vi "LoadObjects_LookupTable.vi"(6 "UIMsgReg.":bool, 8 "error in (no error)":errorcluster, 9 "UIMsg":refnum<class "SendMessage.lvclass">, 10 "sub-system cfgs":T1[](array[typedef])) -> (0 "error out":errorcluster, 3 "sub-systems out":refnum<class "sub-systems.lvclass">)   [LabVIEW 2019, in "sub-systems.lvclass"]
uses:
  sub-systems.lvclass
  VXMCfg/sub-syst.n.ctl
  SendMessage/SendMessage.lvclass
  sub-systems.lvclass/sub-systems.ctl
  Support/MessageAPI/UIMessage.ctl
  VSMx2/VXMx2.lvclass
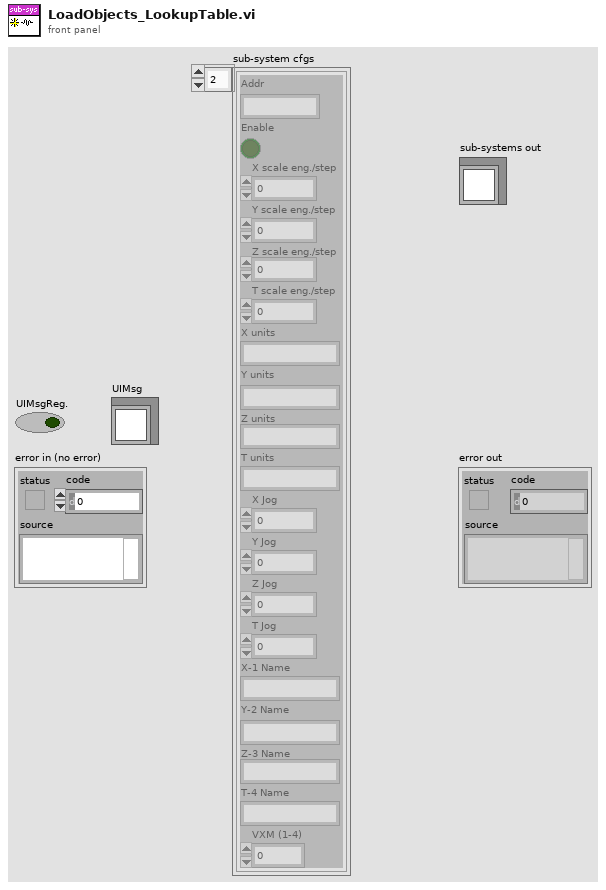
[diagram p1: front panel]
types:
  T1 = typedef "sub-syst.n.ctl" = cluster{"Addr":string, "Enable":bool, "X scale eng./step":dbl, "Y scale eng./step":dbl, "Z scale eng./step":dbl, "T scale eng./step":dbl, "X units":string, "Y units":string, "Z units":string, "T units":string, "X Jog":dbl, "Y Jog":dbl, "Z Jog":dbl, "T Jog":dbl, "X-1 Name":string, "Y-2 Name":string, "Z-3 Name":string, "T-4 Name":string, "VXM (1-4)":i32}
  T2 = typedef "UIMessage.ctl" = cluster{"EventCode":i32, "Numeric":dbl, "String":string, "Variant":variant}
  T3 = cluster{"mmWaveName":string, "Sub-syst":i32, "Axis":string}[]
  T4 = cluster{"mmWaveName":string, "Sub-syst":i32, "Axis":string}
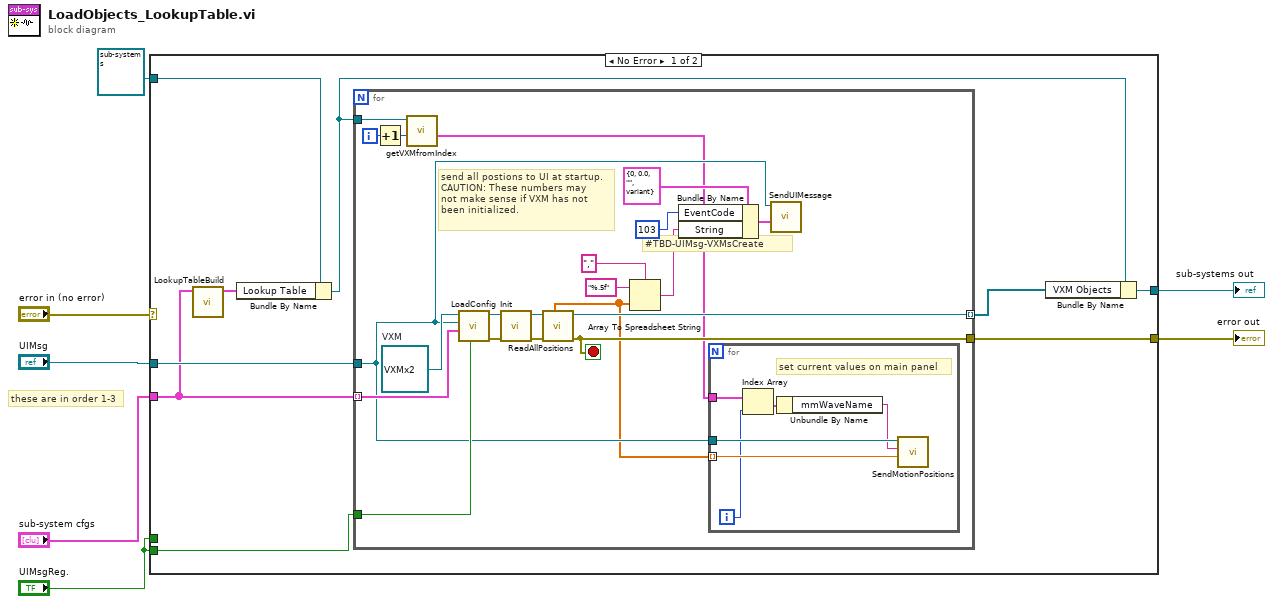
[diagram p0: block diagram]
diagram:
  # "these are in order 1-3"
  n1 = case shown="No Error" "error in (no error)" {
    selector: "error in (no error)" -> [_ w45]
    tunnel: [w12 w45] -> w6
    tunnel: [w14 w44] -> w4
    tunnel: refnum<class "sub-systems.lvclass"> refnum ("sub-systems in") -> [w11 w44]
    tunnel: "sub-system cfgs" -> [w9 _]
    tunnel: "UIMsg" -> [w16 _]
    tunnel: "UIMsgReg." -> [_ _]
    tunnel: "UIMsgReg." -> [w15 _]
    frame No Error {
      n2 = call "LookupTableBuild.vi"("sub-system cfgs"=w9) -> ("Lookup Table"=w8:T3)  [unwired: 10 in]
      n3 = Bundle By Name(cluster=w11, "Lookup Table"=w8) -> (w10:refnum<class "sub-systems.lvclass">)
      n4 = for {
        tunnel: [w27] -> w12
        tunnel: [w26] -> w13 mode=indexing
        tunnel: w9 -> [w24] mode=indexing
        tunnel: w16 -> [w22]
        tunnel: w15 -> [w23]
        tunnel: w10 -> [w20]
        i -> [w19]
        stop <- w27 stop-if-true
        w28 = refnum<class "VXMx2.lvclass"> refnum  # VXM
        # "send all postions to UI at startup.\nCAUTION: These numbers may\nnot make sense if VXM has not\nbeen initialized."
        # "#TBD-UIMsg-VXMsCreate"
        n5 = Increment(x=w19) -> (x+1=w18:i32)
        n6 = call "getVXMfromIndex.vi"("Subsystem 1, 2, 3"=w18, "sub-systems in"=w20) -> ("All Axes this subsystem"=w17:T3)  [unwired: 5 in, 4 out]
        n7 = call "LoadConfig.vi"("UIMsgReg."=w23, "sub-syst Cfg"=w24, "UIMsg"=w22, "VXMx2 in"=w28) -> ("error out"=w29:errorcluster, "VXMx2 out"=w30:refnum<class "VXMx2.lvclass">)  [unwired: 6 in]
        n8 = call "Init.vi"("error in (no error)"=w29, "VXMx2 in"=w30) -> ("error out"=w32:errorcluster, "VXMx2 out"=w31:refnum<class "VXMx2.lvclass">)  [unwired: 8 in]
        n9 = call "ReadAllPositions.vi"("error in (no error)"=w32, "VXMx2 in"=w31) -> ("error out"=w27:errorcluster, "VXMx2 out"=w26:refnum<class "VXMx2.lvclass">, "All Positions, eng units"=w21:dbl[])  [unwired: 2 in, 5 out]
        n10 = Array To Spreadsheet String(delimiter (Tab)=",", array=w21, 3:"%.5f" ("format string")) -> (spreadsheet string=w37:string)
        n11 = Bundle By Name(cluster=T2 {"EventCode"=0, "Numeric"=0.0, "String"="", "Variant"=variant} ("UIMsg"), "EventCode"=103, "String"=w37) -> (w25:T2)
        n12 = for {
          tunnel: w22 -> [w42]
          tunnel: w21 -> [w43] mode=indexing
          tunnel: w17 -> [w39]
          i -> [w41]
          # "set current values on main panel"
          n13 = Index Array(array=w39, index=w41) -> (element=w40:T4)
          n14 = Unbundle By Name(w40) -> ("mmWaveName"=w38:string)
          n15 = call "SendMotionPositions.vi"("Axis Position, eng."=w43, "mmWave Axis Name"=w38, "SendMessage in"=w42) -> ()  [unwired: 7 in, 2 out]
        }
        n16 = call-dynamic "SendUIMessage.vi"("UIMsg"=w25, "SendMessage in"=w22) -> ()  [unwired: 8 in, 2 out]
      }
      n17 = Bundle By Name(cluster=w10, "VXM Objects"=w13) -> (w14:refnum<class "sub-systems.lvclass">)
    }
    frame Error {
    }
  }
  "error out" <- w6
  "sub-systems out" <- w4
